vi "DB_Historicos.vi"(8 "error in (no error)":errorcluster, 9 "Final":timestamp, 10 "Inicio":timestamp, 11 "ID_EQUIPO":i32=1) -> (0 "error out":errorcluster, 3 "Data":string[][](array[string]))   [LabVIEW 2018]
uses:
  <vilib>/addons/database/Connection.llb/DB Tools Open Connec (Path).vi
  <vilib>/addons/database/Connection.llb/Conn Execute.vi
  <vilib>/addons/database/Recordset.llb/Rec Fetch Recordset Data (R).vi
  <vilib>/addons/database/Recordset.llb/Rec Destroy - Connection.vi
  <vilib>/addons/database/_DB Variant To Data/Database Variant To Data.xnode
  <vilib>/addons/database/NI_Database_API.lvlib
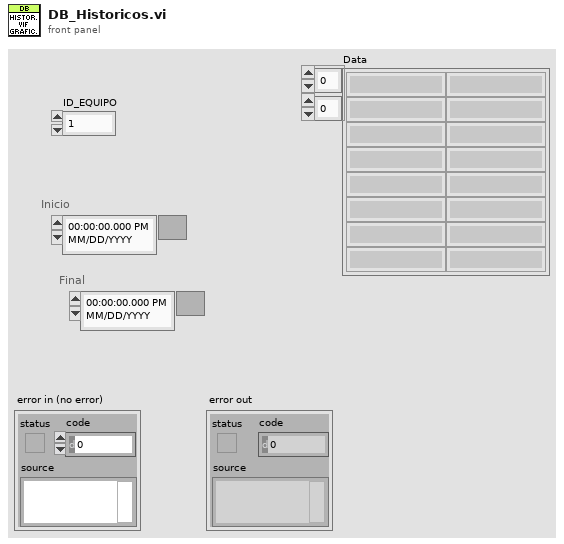
[diagram p1: front panel]
types:
  T1 = typedef "NI_Database_API.lvlib/Conn ObjectReference.ctl" = refnum<k1>
  T2 = typedef "NI_Database_API.lvlib/Rec ObjectReference.ctl" = refnum<k1>
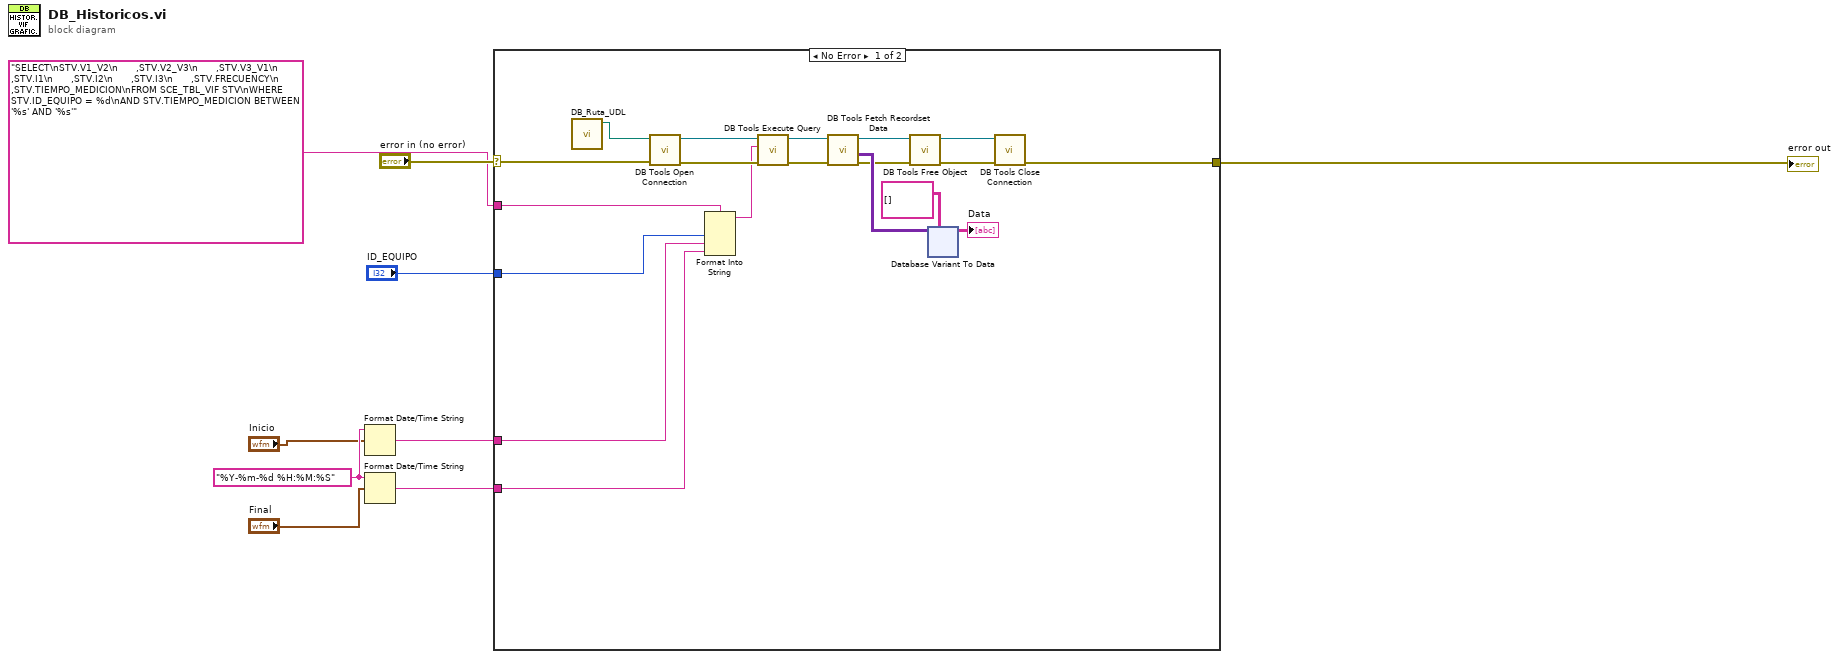
[diagram p0: block diagram]
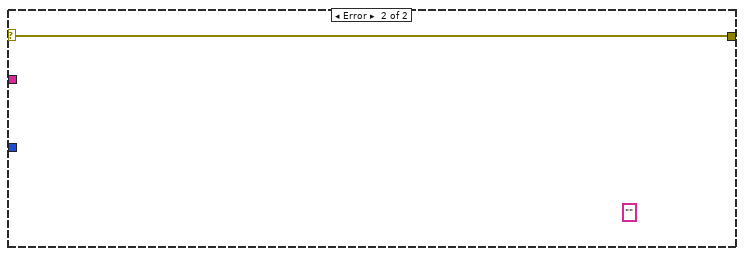
[diagram p2: hidden frame]
diagram:
  w5 = "%Y-%m-%d %H:%M:%S" ("time format string (%c)")
  n1 = Format Date/Time String(time format string (%c)=w5, seconds (now)="Inicio") -> (date/time string=w2:string)  [unwired: 1 in]
  n2 = Format Date/Time String(time format string (%c)=w5, seconds (now)="Final") -> (date/time string=w1:string)  [unwired: 1 in]
  n3 = case shown="No Error" "error in (no error)" {
    selector: "error in (no error)" -> [w23 w73]
    tunnel: [w25 w73] -> w8
    tunnel: "SELECT\nSTV.V1_V2\n      ,STV.V2_V3\n      ,STV.V3_V1\n      ,STV.I1\n      ,STV.I2\n      ,STV.I3\n      ,STV.FRECUENCY\n      ,STV.TIEMPO_MEDICION\nFROM SCE_TBL_VIF STV\nWHERE STV.ID_EQUIPO = %d\nAND STV.TIEMPO_MEDICION BETWEEN '%s' AND '%s'" ("SQL") -> [w15 _]
    tunnel: "ID_EQUIPO" -> [w17 _]
    tunnel: w2 -> [w13 _]
    tunnel: w1 -> [w12 _]
    frame No Error {
      n4 = call "DB_Ruta_UDL.vi"() -> ("UDL ruta"=w11:path)  [unwired: 11 in]
      n5 = call-poly <vilib>:"DB Tools Open Connection.vi"("error in (no error)"=w23, "connection information"=w11) -> ("error out"=w28:errorcluster, "connection reference"=w26:T1)  [unwired: 6 in]
      n6 = Format Into String(format string=w15, w17, w13, w12) -> (resulting string=w14:string)  [unwired: 2 in, 1 out]
      n7 = call-poly <vilib>:"DB Tools Execute Query.vi"("error in (no error)"=w28, "SQL query"=w14, "connection reference"=w26) -> ("error out"=w24:errorcluster, "recordset reference"=w22:T2)  [unwired: 5 in]
      n8 = call-poly <vilib>:"DB Tools Fetch Recordset Data.vi"("error in (no error)"=w24, "recordset reference"=w22) -> ("error out"=w18:errorcluster, "recordset data"=w19:variant[][], "recordset reference out"=w21:T2)  [unwired: 3 in]
      n9 = call-poly <vilib>:"DB Tools Free Object.vi"("error in (no error)"=w18, "recordset reference"=w21) -> ("error out"=w27:errorcluster, "connection reference"=w10:T1)  [unwired: 8 in]
      n10 = xnode "Database Variant To Data"("database variant"=w19, "type"=string[][] []) -> ("data"=→"Data":string[][])  [unwired: 1 in, 1 out]
      n11 = call <vilib>:"DB Tools Close Connection.vi"("error in (no error)"=w27, "connection reference"=w10) -> ("error out"=w25:errorcluster)  [unwired: 5 in]
    }
    frame Error {
      (unwired) ""
    }
  }
  "error out" <- w8
